vi "Pre_Loop_Initialization_FGV.vi"(8 "error in (no error)":errorcluster, 10 "DUT":string, 11 "VI in":refnum<vi>) -> (0 "error out":errorcluster, 2 "queue Out":refnum<queue>, 3 "User Event out":refnum<user-event>)   [LabVIEW 2024, in "Relay_Module.lvlib"]
doc: "This VI\n------------------------------------------------\nPer_Loop_Initialize\n------------------------------------------------\n-Generate the Communication Queue Reference with FGV.\n-Get the Common User Events Reference at Application Level."
uses:
  Relay_Module.lvlib
  UserEvents/Controls/User_Events_Action_Control.ctl
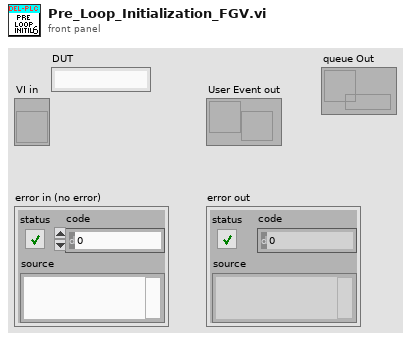
[diagram p1: front panel]
types:
  T1 = typedef "Relay_Module.lvlib/User_Events_Action_Control.ctl" = enum16{"Get", "Create", "Destroy"}
  T2 = cluster{"Message":string, "Message Data":variant}
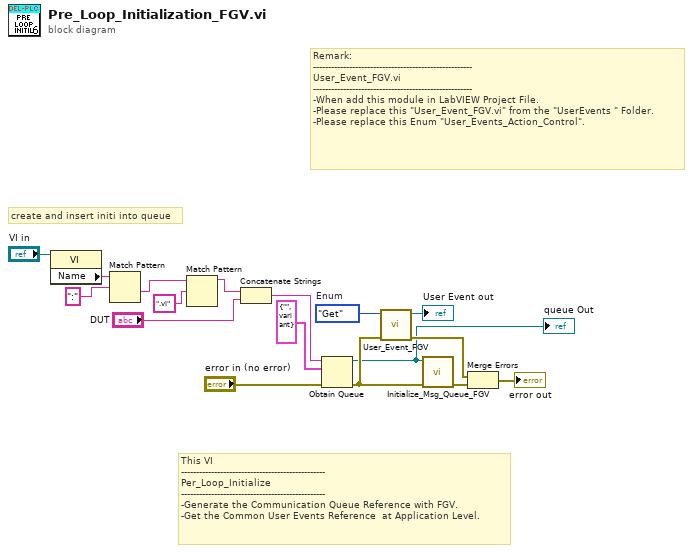
[diagram p0: block diagram]
diagram:
  w12 = User_Events_Action_Control."Get"  # Enum
  # "Remark:\n-----------------------------------------------------\nUser_Event_FGV.vi\n-----------------------------------------------------\n-When add this module in LabVIEW Project File.\n-Please replace this \"User_Event_FGV.vi\" from the \"UserEvents \" Folder.\n-Please replace this Enum \"User_Events_Action_Control\"."
  # "This VI\n------------------------------------------------\nPer_Loop_Initialize\n------------------------------------------------\n-Generate the Communication Queue Reference with FGV.\n-Get the Common User Events Reference  at Application Level."
  # "create and insert initi into queue"
  n1 = property class="VI"(reference="VI in") -> ("Name"=w7:string)  [unwired: 1 in, 2 out]
  n2 = Match Pattern(string=w7, regular expression=":") -> (after substring=w3:string)  [unwired: 1 in, 3 out]
  n3 = Match Pattern(string=w3, regular expression=".vi") -> (before substring=w1:string)  [unwired: 1 in, 3 out]
  n4 = Concatenate Strings(w1, "DUT") -> (w5:string)
  n5 = Obtain Queue(name (unnamed)=w5, element data type=T2 {"Message"="", "Message Data"=variant} ("Message Cluster"), error in (no error)="error in (no error)") -> (queue out=w11:refnum<queue>, error out=w13:errorcluster)  [unwired: 2 in, 1 out]
  "queue Out" <- w11
  n6 = call "User_Event_FGV.vi"("error in (no error)"=w13, "Enum"=w12) -> ("error out"=w15:errorcluster, "User Event out"=→"User Event out":refnum<user-event>)  [unwired: 8 in]
  n7 = call "Initialize_Msg_Queue_FGV.vi"("error in (no error)"=w13, "queue IN"=w11) -> ("error out"=w16:errorcluster)  [unwired: 9 in]
  n8 = Merge Errors(w15, w16) -> (→"error out":errorcluster)
